vi "GetGraphTypeInfo.vi"(0 "reference in":refnum<class "Graph.lvclass">, 5 "error in (no error)":errorcluster) -> (14 "reference out":refnum<class "Graph.lvclass">, 15 "GraphTypeName":string, 16 "NodeTypes":refnum<class "AbstractNode.lvclass">[](array[class]), 17 "EdgeTypes":refnum<class "AbstractEdge.lvclass">[](array[class]), 18 "GraphTypeUserName":string, 19 "error out":errorcluster)   [LabVIEW 2014, in "Graph.lvclass"]
uses:
  <resource>/Framework/Providers/Open_GDS/UML/Graph_class/Graph.lvclass
  <resource>/Framework/Providers/Open_GDS/UML/AbstractNode_class/AbstractNode.lvclass
  <resource>/Framework/Providers/Open_GDS/UML/AbstractEdge_class/AbstractEdge.lvclass
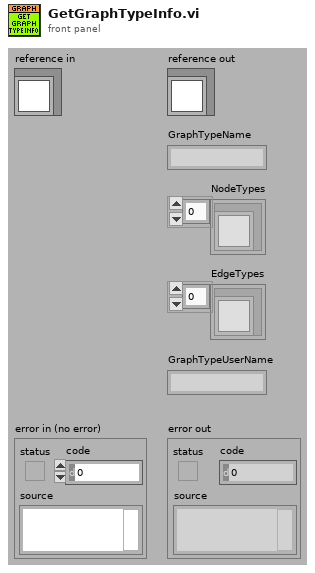
[diagram p1: front panel]
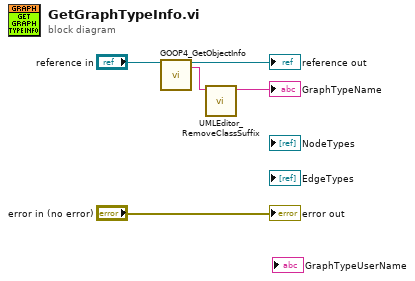
[diagram p0: block diagram]
diagram:
  n1 = call <vilib>:"GOOP4_GetObjectInfo.vi"("ObjectIn"="reference in") -> ("ObjectOut"=→"reference out":refnum<class "Graph.lvclass">, "ObjectRuntimeClassName"=w2:string)  [unwired: 13 in, 4 out]
  n2 = call <resource>:"UMLEditor_RemoveClassSuffix.vi"("ObjectRuntimeClassName in"=w2) -> ("ObjectRuntimeClassName out"=→"GraphTypeName":string)  [unwired: 10 in]
  "error out" <- "error in (no error)"
